vi "dosimat_fill_ii.vi"(1 "Dosimat Port In":refnum<visa-resource-name>="COM1") -> ()   [LabVIEW 2010]
panel:
  out "Dosimat Port Out":refnum<visa-resource-name>="COM1"
  in  "error in":errorcluster
  out "error out":errorcluster
  # "mooseNote: tell the Dosimat to fill... before this gets called\nthe vent relay (4) needs to be opened. And then\nclosed afterwards."
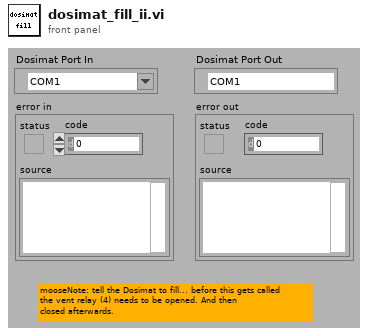
[diagram p1: front panel]
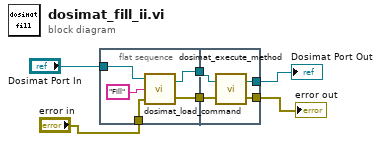
[diagram p0: block diagram]
diagram:
  n1 = flat-sequence {
    tunnel: [w9] -> w6
    tunnel: "Dosimat Port In" -> [w11]
    tunnel: [w8] -> w4
    tunnel: "error in" -> [w7]
    tunnel: w6 -> [w15]
    tunnel: w4 -> [w14]
    tunnel: [w13] -> w2
    tunnel: [w12] -> w1
    frame #0 {
      n2 = call "dosimat_load_command.vi"("error in"=w7, "Method"="Fill", "Dosimat Port In"=w11) -> ("error out"=w8:errorcluster, "Dosimat Port Out"=w9:refnum<visa-resource-name>)
    }
    frame #1 {
      n3 = call "dosimat_execute_method.vi"("error in"=w14, "Dosimat Port In"=w15) -> ("error out"=w13:errorcluster, "Dosimat Port Out"=w12:refnum<visa-resource-name>)
    }
  }
  "error out" <- w2
  "Dosimat Port Out" <- w1
